vi "Write folders.vi"(8 "error in (no error)":errorcluster, 10 "Parameters":T1[](array[typedef])=[{"name"="AI.AI", "data type"=111, "access level"=enum."read-only", "description"="AI Value Array", "period"=enum."500 ms"}, {"name"="AI.AI_ALRState", "data type"=106, "access level"=enum."read-only", "description"="AI ALR State Array", "period"=enum."500 ms"}, {"name"="AI.AI_Descriptions", "data type"=112, "access level"=enum."read-only", "description"="AI Descriptions Array", "period"=enum."on_load"}, {"name"="AI.AI_Names", "data type"=112, "access level"=enum."read-only", "description"="AI Names Array", "period"=enum."500 ms"}, {"name"="AI.AI_State", "data type"=106, "access level"=enum."read-only", "description"="AI State Array", "period"=enum."500 ms"}, {"name"="ALR.ALR", "data type"=101, "access level"=enum."read-only", "description"="ALARM Array", "period"=enum."100 ms"}, {"name"="ALR.ALR_Block", "data type"=101, "access level"=enum."read-only", "description"="ALR Blocked Array", "period"=enum."100 ms"}, {"name"="ALR.ALR_Descriptions", "data type"=112, "access level"=enum."read-only", "description"="ALR Descriptions Array", "period"=enum."on_load"}, {"name"="ALR.ALR_Names", "data type"=112, "access level"=enum."read-only", "description"="ALR Names Array", "period"=enum."100 ms"}, {"name"="ALR.ALR_Pcode", "data type"=112, "access level"=enum."read-only", "description"="ALR Param Names Array", "period"=enum."on_load"}, {"name"="ALR.ALR_State", "data type"=106, "access level"=enum."read-only", "description"="ALR State Array", "period"=enum."100 ms"}, {"name"="AO.AO", "data type"=111, "access level"=enum."read-only", "description"="AO Value Array", "period"=enum."500 ms"}, {"name"="AO.AO_ALRState", "data type"=106, "access level"=enum."read-only", "description"="AO ALR State Array", "period"=enum."500 ms"}, {"name"="AO.AO_Descriptions", "data type"=112, "access level"=enum."read-only", "description"="AO Descriptions Array", "period"=enum."on_load"}, {"name"="AO.AO_Names", "data type"=112, "access level"=enum."read-only", "description"="AO Names Array", "period"=enum."500 ms"}, {"name"="AO.AO_State", "data type"=106, "access level"=enum."read-only", "description"="AO State Array", "period"=enum."500 ms"}, {"name"="DI.DI", "data type"=101, "access level"=enum."read-only", "description"="DI Value Array", "period"=enum."100 ms"}, {"name"="DI.DI_ALRState", "data type"=106, "access level"=enum."read-only", "description"="DI ALR State Array", "period"=enum."100 ms"}, {"name"="DI.DI_Descriptions", "data type"=112, "access level"=enum."read-only", "description"="DI Descriptions Array", "period"=enum."on_load"}, {"name"="DI.DI_Names", "data type"=112, "access level"=enum."read-only", "description"="DI Names Array", "period"=enum."100 ms"}, {"name"="DI.DI_State", "data type"=106, "access level"=enum."read-only", "description"="DI State Array", "period"=enum."100 ms"}, {"name"="DO.DO", "data type"=101, "access level"=enum."read-only", "description"="DO Value Array", "period"=enum."100 ms"}, {"name"="DO.DO_ALRState", "data type"=106, "access level"=enum."read-only", "description"="DO ALR State Array", "period"=enum."100 ms"}, {"name"="DO.DO_Descriptions", "data type"=112, "access level"=enum."read-only", "description"="DO Descriptions Array", "period"=enum."on_load"}, {"name"="DO.DO_Names", "data type"=112, "access level"=enum."read-only", "description"="DO Names Array", "period"=enum."100 ms"}, {"name"="DO.DO_State", "data type"=106, "access level"=enum."read-only", "description"="DO State Array", "period"=enum."100 ms"}, {"name"="HT1.control", "data type"=12, "access level"=enum."none", "description"="HT1 reg input", "period"=enum."100 ms"}, {"name"="HT1.state", "data type"=12, "access level"=enum."read-only", "description"="HT1 reg output", "period"=enum."100 ms"}, {"name"="HT2.control", "data type"=12, "access level"=enum."none", "description"="HT2 reg input", "period"=enum."100 ms"}, {"name"="HT2.state", "data type"=12, "access level"=enum."read-only", "description"="HT2 reg output", "period"=enum."100 ms"}] {"data type" items=["Boolean"=1, "SByte"=2, "Byte"=3, "Int16"=4, "UInt16"=5, "Int32"=6, "UInt32"=7, "Int64"=8, "UInt64"=9, "Float"=10, "Double"=11, "String"=12, "DateTime"=13, "ByteString"=15, "Array of Boolean"=101, "Array of SByte"=102, "Array of Byte"=103, "Array of Int16"=104, "Array of UInt16"=105, "Array of Int32"=106, "Array of UInt32"=107, "Array of Int64"=108, "Array of UInt64"=109, "Array of Float"=110, "Array of Double"=111, "Array of String"=112, "Array of DateTime"=113, "Array of ByteString"=115, "Matrix of Boolean"=201, "Matrix of SByte"=202, "Matrix of Byte"=203, "Matrix of Int16"=204, "Matrix of UInt16"=205, "Matrix of Int32"=206, "Matrix of UInt32"=207, "Matrix of Int64"=208, "Matrix of UInt64"=209, "Matrix of Float"=210, "Matrix of Double"=211, "Matrix of String "=212, "Matrix of DateTime"=213, "Matrix of ByteString"=215]}, 11 "OPC UA server refnum in":T6) -> (0 "error out":errorcluster, 2 "Folders":T5[](array[typedef]), 3 "OPC UA server refnum out":T6)   [LabVIEW 2019, in "OPC addons.lvlib"]
uses:
  OPC addons.lvlib
  <vilib>/OPCUA/controls/OPC UA Server Refnum.ctl
  <vilib>/OPCUA/controls/NodeId.ctl
  OPC tag.ctl
  <vilib>/OPCUA/controls/Data Type.ctl
  Access level.ctl
  Period.ctl
  <vilib>/OPCUA/NI OPC UA Server.lvlib
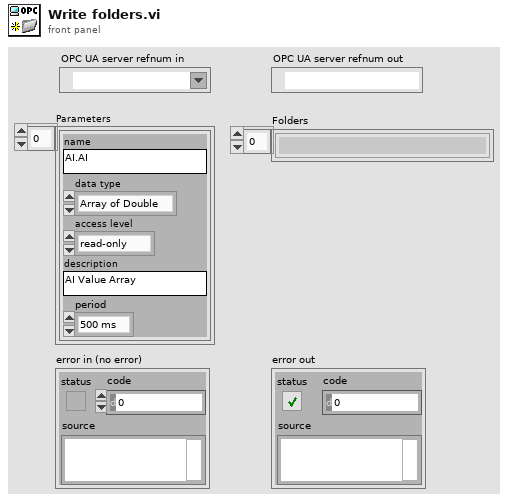
[diagram p1: front panel]
types:
  T1 = typedef "OPC addons.lvlib/OPC tag.ctl" = cluster{"name":string, "data type":T2, "access level":T3, "description":string, "period":T4}
  T2 = typedef "Data Type.ctl" = u16
  T3 = typedef "OPC addons.lvlib/Access level.ctl" = enum16{"none", "read-only", "write-only", "read/write"}
  T4 = typedef "OPC addons.lvlib/Period.ctl" = enum16{"on_load", "100 ms", "500 ms", "1 s"}
  T5 = typedef "NodeId.ctl" = string
  T6 = typedef "OPC UA Server Refnum.ctl" = refnum<k21>
  T7 = cluster{"name":string, "data type":T2, "access level":u16, "description":string}
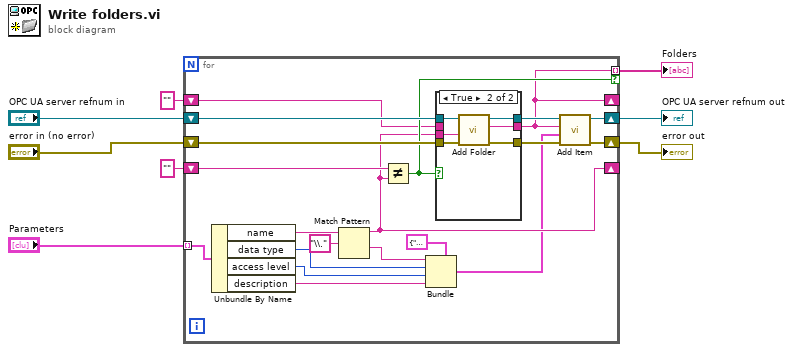
[diagram p0: block diagram]
diagram:
  n1 = for {
    tunnel: [w14] -> w3 mode=indexing if=w19
    shift-right: [w23] -> w5
    shift-left: "OPC UA server refnum in" -> [w28]
    shift-right: [w24] -> w4
    shift-left: "error in (no error)" -> [w27]
    tunnel: "Parameters" -> [w22] mode=indexing
    shift-right: [w15] -> _
    shift-left: "" ("name") -> [w20]
    shift-right: [w14] -> _
    shift-left: T5 "" ("folder node ID") -> [w13]
    n2 = Unbundle By Name(w22) -> ("name"=w18:string, "data type"=w16:T2, "access level"=w9:T3, "description"=w10:string)
    n3 = Match Pattern(string=w18, regular expression="\\.") -> (before substring=w15:string, after substring=w17:string)  [unwired: 1 in, 2 out]
    n4 = Not Equal?(x=w20, y=w15) -> (x != y?=w19:bool)
    n5 = Bundle(cluster=T7 {"name"="", "data type"=1, "access level"=3, "description"=""} ("item"), "name"=w17, "data type"=w16, "access level"=w9, "description"=w10) -> (w11:T7)
    n6 = case shown="True" w19 {
      tunnel: w28 -> [w31 w37]
      tunnel: w27 -> [w30 w36]
      tunnel: [w31 w35] -> w26
      tunnel: [w29 w34] -> w14
      tunnel: [w30 w33] -> w25
      tunnel: w15 -> [_ w32]
      tunnel: w13 -> [w29 _]
      frame False {
      }
      frame True {
        n7 = call <vilib>:"Add Folder.vi"("error in (no error)"=w36, "folder name"=w32, "OPC UA server refnum in"=w37) -> ("error out"=w33:errorcluster, "folder node ID"=w34:T5, "OPC UA server refnum out"=w35:T6)  [unwired: 5 in]
      }
    }
    n8 = call <vilib>:"Add Item.vi"("error in (no error)"=w25, "item"=w11, "parent folder node ID"=w14, "OPC UA server refnum in"=w26) -> ("error out"=w24:errorcluster, "OPC UA server refnum out"=w23:T6)  [unwired: 3 in, 2 out]
  }
  "OPC UA server refnum out" <- w5
  "error out" <- w4
  "Folders" <- w3
